vi "Read configuration.vi"(8 "error in (no error)":errorcluster, 11 "Thermo Instrument in":refnum<class "Thermo Instrument.lvclass">) -> (0 "error out":errorcluster, 2 "configuration":refnum<class "CEF_serializable configuration.lvclass">, 3 "Thermo Instrument out":refnum<class "Thermo Instrument.lvclass">)   [LabVIEW 2025, in "Thermo.lvlib" / "Thermo Instrument.lvclass"]
uses:
  Thermo Instrument.lvclass
  Users/Public/Documents/Sandia National Labs/TSS Plugin/CEF.lvlibp/serializable configuration/CEF_serializable configuration.lvclass
  Thermo Instrument.lvclass/Thermo Instrument.ctl
  Thermo configuration/Thermo configuration.lvclass
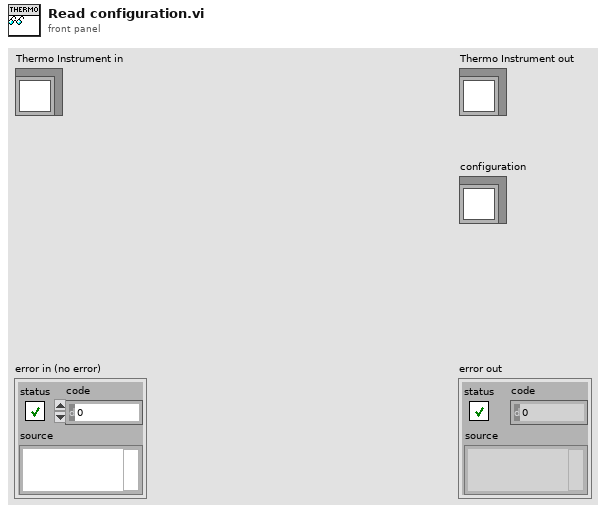
[diagram p1: front panel]
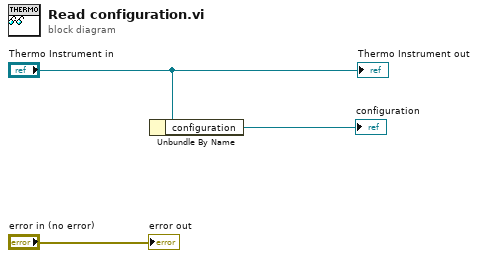
[diagram p0: block diagram]
diagram:
  n1 = Unbundle By Name("Thermo Instrument in") -> ("configuration"=→"configuration":refnum<class "Thermo configuration.lvclass">)
  "error out" <- "error in (no error)"
  "Thermo Instrument out" <- "Thermo Instrument in"
